vi "createCanFile.vi"(8 "error in":errorcluster, 11 "contentArray":string[](array[string])) -> (0 "error out":errorcluster)   [LabVIEW 2010]
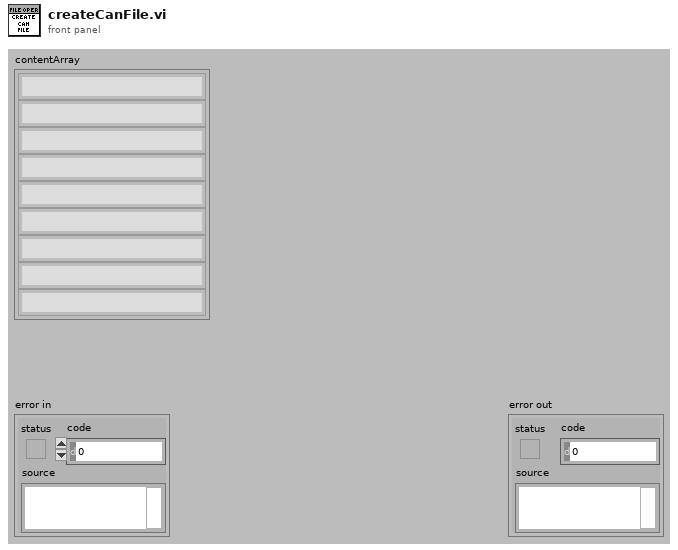
[diagram p1: front panel]
types:
  T1 = enum16{"open", "replace", "create", "open or create", "replace or create", "replace or create with confirmation"}
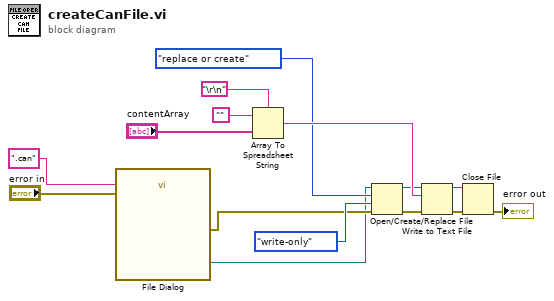
[diagram p0: block diagram]
diagram:
  n1 = call "File Dialog"("default name"=".can" ("prompt"), "error in"="error in") -> ("selected path"=w2:path, "error out"=w4:errorcluster)  [unwired: 10 in, 2 out]
  n2 = Array To Spreadsheet String(delimiter (Tab)="\r\n", array="contentArray", 3:"") -> (spreadsheet string=w10:string)
  n3 = Open/Create/Replace File(file path (use dialog)=w2, error in=w4, operation (0:open)=T1."replace or create", access (0:read/write)=enum16{"read/write", "read-only", "write-only"}."write-only") -> (refnum out=w9:refnum<file>, error out=w11:errorcluster)  [unwired: 2 in, 1 out]
  n4 = Write to Text File(file (use dialog)=w9, text=w10, error in=w11) -> (refnum out=w13:refnum<file>, error out=w14:errorcluster)  [unwired: 1 in, 1 out]
  n5 = Close File(refnum=w13, error in=w14) -> (error out=→"error out":errorcluster)  [unwired: 1 out]
